vi "Abort Scan.vi"(0 "Notifier Name":string, 11 "Error In":errorcluster) -> (4 "Notifier Name Dup":string, 8 "Success":bool, 15 "Error Out":errorcluster)   [LabVIEW 2020]
uses:
  3 Mirror Scan Type Defs/3 Mirror Scan Note Type.ctl
  3 Mirror Scan Type Defs/3 Mirror Scan Actions.ctl
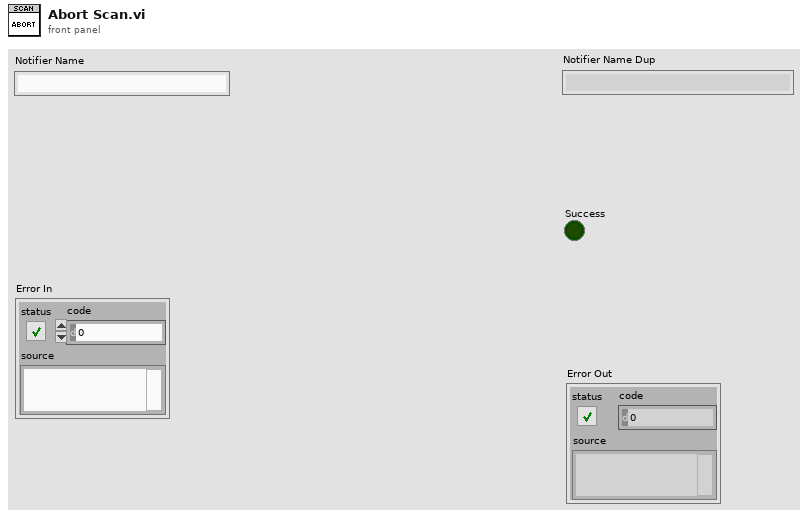
[diagram p1: front panel]
types:
  T1 = typedef "3 Mirror Scan Note Type.ctl" = cluster{"Actions":T2, "Global Rectangle":i32[], "Running":bool, "Scan Frequency (Hz)":dbl, "Scan Time (s)":dbl}
  T2 = typedef "3 Mirror Scan Actions.ctl" = enum16{"Idle", "Scan Timed", "Scan Live", "Convert ROI", "Run Scan", "Exit Loop", "Quit"}
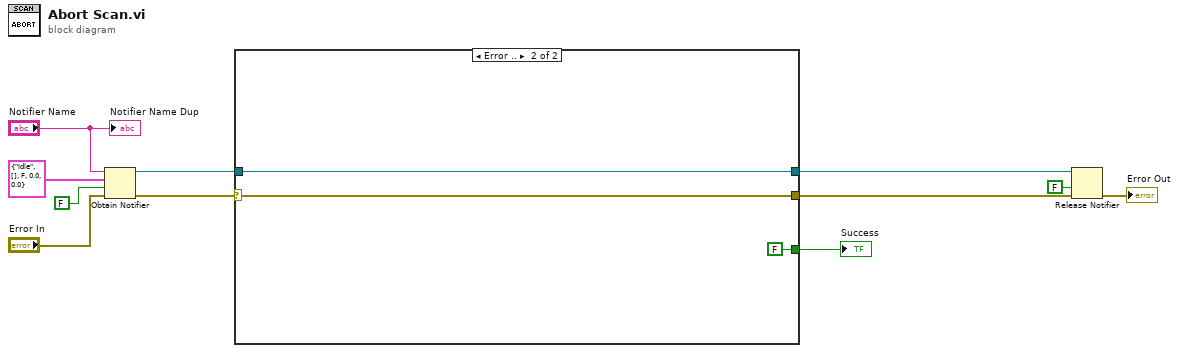
[diagram p0: block diagram]
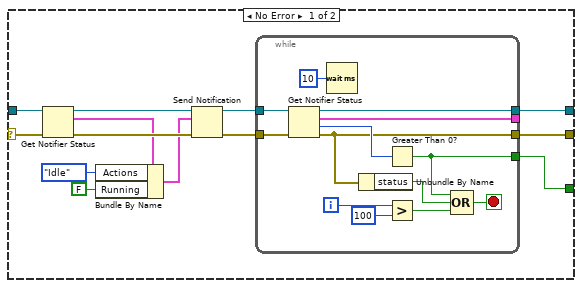
[diagram p2: hidden frame]
diagram:
  n1 = Obtain Notifier(name (unnamed)="Notifier Name", notification data type=T1 {"Actions"=enum."Idle", "Global Rectangle"=[], "Running"=FALSE, "Scan Frequency (Hz)"=0.0, "Scan Time (s)"=0.0} ("3 Mirror Notifier"), create if not found? (T)=FALSE, error in (no error)="Error In") -> (notifier out=w7:refnum<notifier>, error out=w8:errorcluster)  [unwired: 1 out]
  n2 = case shown="Error .." w8 {
    selector: w8 -> [w23 w39]
    tunnel: w7 -> [w24 w40]
    tunnel: [w14 w40] -> w5
    tunnel: [w13 w39] -> w3
    tunnel: [w12 FALSE] -> w1
    frame No Error {
      n3 = Get Notifier Status(notifier=w24, error in (no error)=w23) -> (notifier out=w22:refnum<notifier>, current notification=w20:T1, error out=w21:errorcluster)  [unwired: 2 out]
      n4 = Bundle By Name(cluster=w20, "Actions"=3_Mirror_Scan_Actions."Idle", "Running"=FALSE) -> (w17:T1)
      n5 = Send Notification(notification=w17, notifier=w22, error in (no error)=w21) -> (notifier out=w16:refnum<notifier>, error out=w15:errorcluster)
      n6 = while {
        tunnel: w16 -> [w37]
        tunnel: w15 -> [w36]
        tunnel: [w28] -> w14
        tunnel: [w27] -> w13
        tunnel: [w26] -> _
        tunnel: [w25] -> w12
        i -> [w34]
        stop <- w29 stop-if-true
        n7 = Get Notifier Status(notifier=w37, error in (no error)=w36) -> (notifier out=w28:refnum<notifier>, current notification=w26:T1, # waiting=w32:i32, error out=w27:errorcluster)  [unwired: 1 out]
        n8 = Wait (ms)(milliseconds to wait=u32 10) -> ()  [unwired: 1 out]
        n9 = Unbundle By Name(w27) -> ("status"=w31:bool)
        n10 = Greater Than 0?(x=w32) -> (x > 0?=w25:bool)
        n11 = Greater?(x=w34, y=100) -> (0:w30:bool)
        n12 = Compound Arithmetic op=OR(w25, w31, w30) -> (w29:bool)
      }
    }
    frame Error {
    }
  }
  "Success" <- w1
  n13 = Release Notifier(notifier=w5, force destroy? (F)=FALSE, error in (no error)=w3) -> (error out=→"Error Out":errorcluster)  [unwired: 2 out]
  "Notifier Name Dup" <- "Notifier Name"
